vi "Decode NTC codes.vi"(11 "NTC Messages":T1(array[cluster])=[{"ID"=1808, "MSGTYPE"=0, "LEN"=8, "DATA[0]"=33, "DATA[1]"=11, "DATA[2]"=56, "DATA[3]"=1, "DATA[4]"=36, "DATA[5]"=0, "DATA[6]"=11, "DATA[7]"=0}, {"ID"=1808, "MSGTYPE"=0, "LEN"=8, "DATA[0]"=34, "DATA[1]"=1, "DATA[2]"=37, "DATA[3]"=0, "DATA[4]"=11, "DATA[5]"=0, "DATA[6]"=1, "DATA[7]"=64}, {"ID"=1808, "MSGTYPE"=0, "LEN"=8, "DATA[0]"=35, "DATA[1]"=0, "DATA[2]"=11, "DATA[3]"=0, "DATA[4]"=1, "DATA[5]"=68, "DATA[6]"=0, "DATA[7]"=11}, {"ID"=1808, "MSGTYPE"=0, "LEN"=8, "DATA[0]"=36, "DATA[1]"=0, "DATA[2]"=1, "DATA[3]"=73, "DATA[4]"=0, "DATA[5]"=11, "DATA[6]"=0, "DATA[7]"=1}, {"ID"=1808, "MSGTYPE"=0, "LEN"=8, "DATA[0]"=37, "DATA[1]"=80, "DATA[2]"=0, "DATA[3]"=11, "DATA[4]"=0, "DATA[5]"=1, "DATA[6]"=86, "DATA[7]"=0}, {"ID"=1808, "MSGTYPE"=0, "LEN"=8, "DATA[0]"=38, "DATA[1]"=11, "DATA[2]"=0, "DATA[3]"=1, "DATA[4]"=89, "DATA[5]"=0, "DATA[6]"=11, "DATA[7]"=0}, {"ID"=1808, "MSGTYPE"=0, "LEN"=8, "DATA[0]"=39, "DATA[1]"=1, "DATA[2]"=104, "DATA[3]"=0, "DATA[4]"=11, "DATA[5]"=0, "DATA[6]"=1, "DATA[7]"=105}, {"ID"=1808, "MSGTYPE"=0, "LEN"=8, "DATA[0]"=40, "DATA[1]"=0, "DATA[2]"=11, "DATA[3]"=0, "DATA[4]"=1, "DATA[5]"=114, "DATA[6]"=0, "DATA[7]"=11}, {"ID"=1808, "MSGTYPE"=0, "LEN"=8, "DATA[0]"=41, "DATA[1]"=0, "DATA[2]"=1, "DATA[3]"=115, "DATA[4]"=0, "DATA[5]"=11, "DATA[6]"=0, "DATA[7]"=1}, {"ID"=1808, "MSGTYPE"=0, "LEN"=8, "DATA[0]"=42, "DATA[1]"=144, "DATA[2]"=0, "DATA[3]"=11, "DATA[4]"=24, "DATA[5]"=1, "DATA[6]"=146, "DATA[7]"=0}, {"ID"=1808, "MSGTYPE"=0, "LEN"=8, "DATA[0]"=43, "DATA[1]"=11, "DATA[2]"=1, "DATA[3]"=0, "DATA[4]"=80, "DATA[5]"=2, "DATA[6]"=8, "DATA[7]"=0}, {"ID"=1808, "MSGTYPE"=0, "LEN"=8, "DATA[0]"=44, "DATA[1]"=0, "DATA[2]"=85, "DATA[3]"=2, "DATA[4]"=8, "DATA[5]"=0, "DATA[6]"=0, "DATA[7]"=176}, {"ID"=1808, "MSGTYPE"=0, "LEN"=8, "DATA[0]"=45, "DATA[1]"=2, "DATA[2]"=8, "DATA[3]"=0, "DATA[4]"=1, "DATA[5]"=96, "DATA[6]"=2, "DATA[7]"=73}, {"ID"=1808, "MSGTYPE"=0, "LEN"=8, "DATA[0]"=46, "DATA[1]"=0, "DATA[2]"=0, "DATA[3]"=0, "DATA[4]"=255, "DATA[5]"=0, "DATA[6]"=0, "DATA[7]"=0}] {"ID" format="%.0x"; "DATA[0]" format="%.0x"; "DATA[1]" format="%.0x"; "DATA[2]" format="%.0x"; "DATA[3]" format="%.0x"; "DATA[4]" format="%.0x"; "DATA[5]" format="%.0x"; "DATA[6]" format="%.0x"; "DATA[7]" format="%.0x"}) -> (2 "NTC codes":u32[](array[numeric]) format="%.0x", 3 "NTCs":string)   [LabVIEW 2025]
panel:
  out "NTC codes1":i32[](array[numeric])
  out "Parameters":i32[](array[numeric]) format="%.0x"
  out "s":i32[](array[numeric]) format="%.0x"
  out "a":i32[](array[numeric])
  out "NTC codes0":i32[](array[numeric]) format="%.0x"
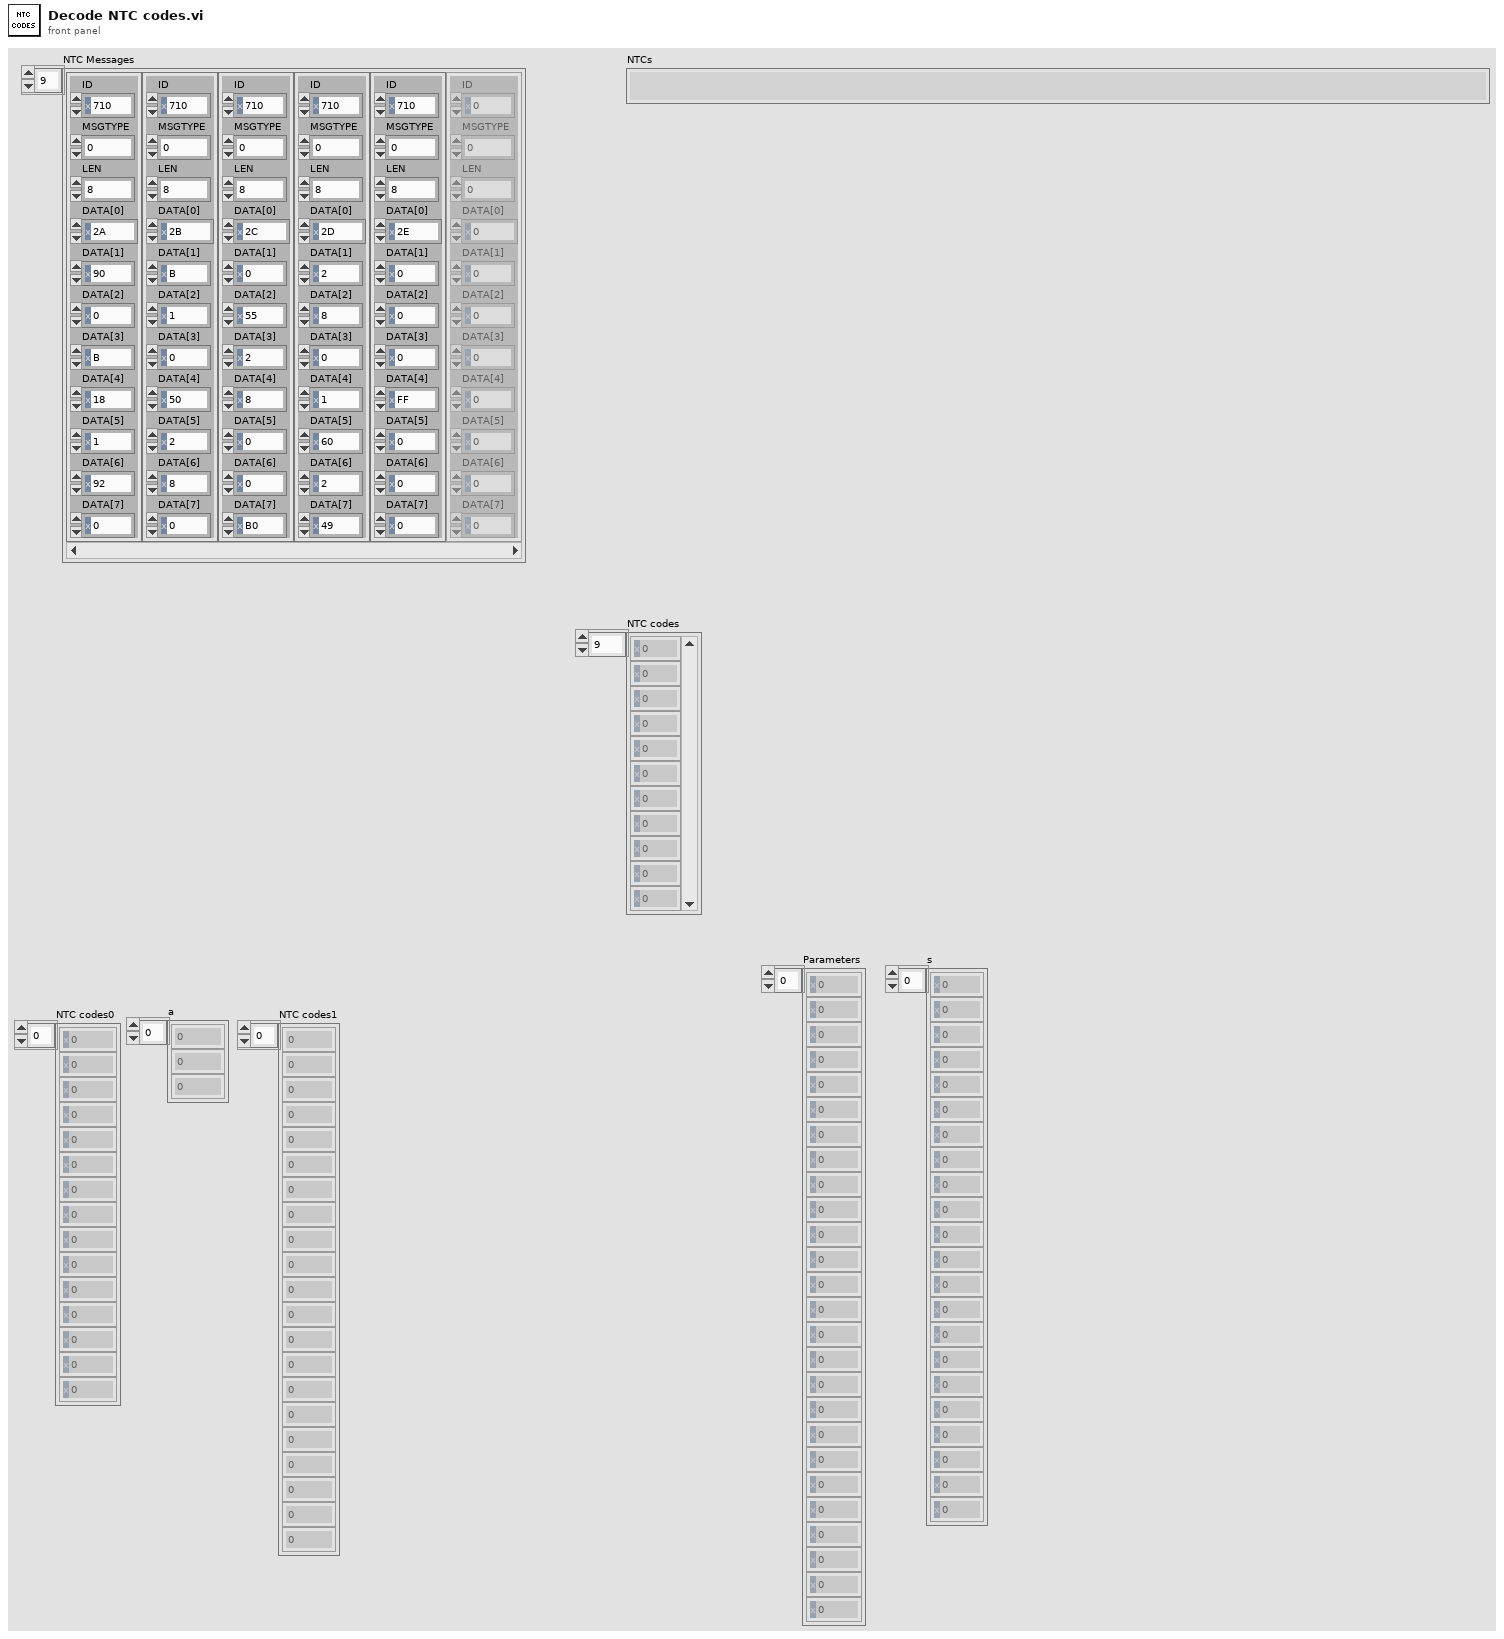
[diagram p1: front panel]
types:
  T1 = cluster{"ID":u32, "MSGTYPE":u8, "LEN":u8, "DATA[0]":u8, "DATA[1]":u8, "DATA[2]":u8, "DATA[3]":u8, "DATA[4]":u8, "DATA[5]":u8, "DATA[6]":u8, "DATA[7]":u8}[]
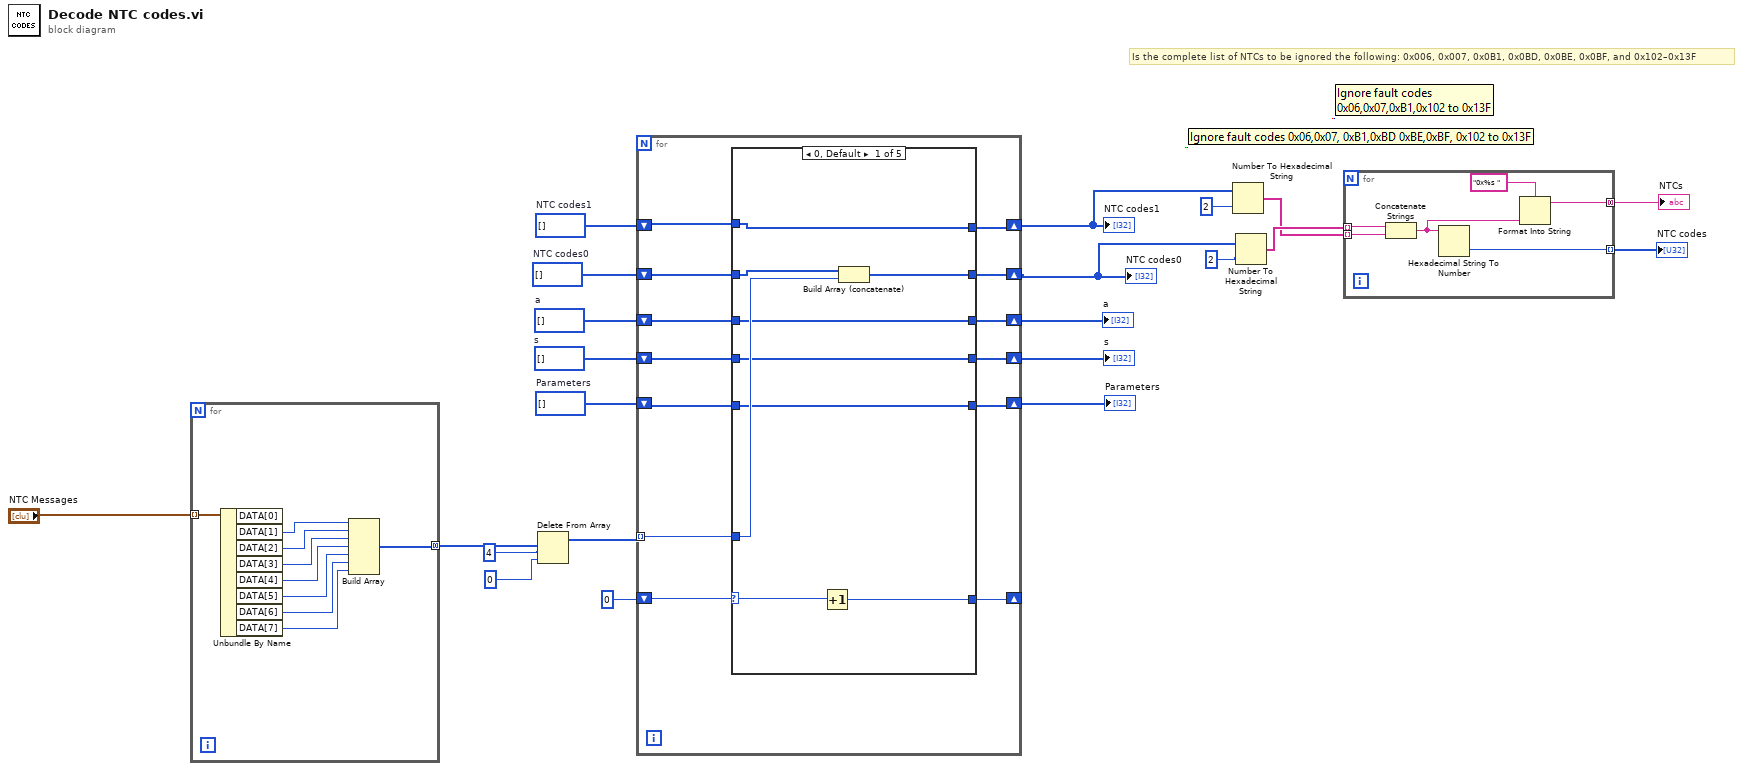
[diagram p0: block diagram]
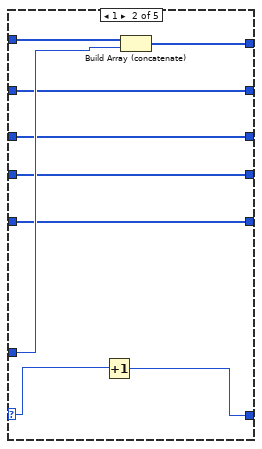
[diagram p2: hidden frame]
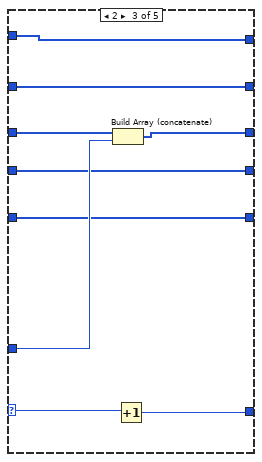
[diagram p3: hidden frame]
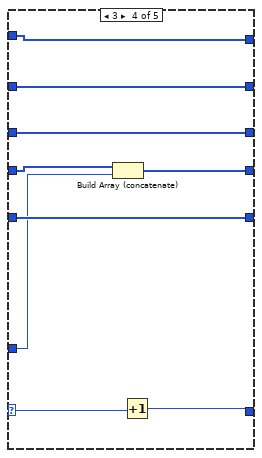
[diagram p4: hidden frame]
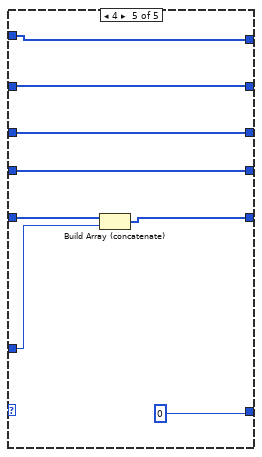
[diagram p5: hidden frame]
diagram:
  w13 = i32[] []  # NTC codes1
  w14 = i32[] []  # Parameters
  w15 = i32[] []  # s
  w16 = i32[] []  # a
  w17 = i32[] []  # NTC codes0
  # "Is the complete list of NTCs to be ignored the following: 0x006, 0x007, 0x0B1, 0x0BD, 0x0BE, 0x0BF, and 0x102–0x13F"
  n1 = for {
    tunnel: "NTC Messages" -> [w31] mode=indexing
    tunnel: [w23] -> w22 mode=concatenating
    n2 = Unbundle By Name(w31) -> ("DATA[1]"=w30:u8, "DATA[2]"=w29:u8, "DATA[3]"=w28:u8, "DATA[4]"=w27:u8, "DATA[5]"=w26:u8, "DATA[6]"=w25:u8, "DATA[7]"=w24:u8)  [unwired: 1 out]
    n3 = Build Array(w30, w29, w28, w27, w26, w25, w24) -> (w23:u8[])
  }
  n4 = Delete From Array(array=w22, length=4, index=0) -> (array with subset deleted=w19:u8[])  [unwired: 1 out]
  n5 = for {
    tunnel: w19 -> [w43] mode=indexing
    shift-right: [w34] -> _
    shift-left: 0 -> [w44]
    shift-right: [w41] -> w7
    shift-left: w17 -> [w42]
    shift-right: [w36] -> w10
    shift-left: w14 -> [w35]
    shift-right: [w37] -> w9
    shift-left: w15 -> [w38]
    shift-right: [w39] -> w11
    shift-left: w16 -> [w40]
    shift-right: [w32] -> w8
    shift-left: w13 -> [w33]
    n6 = case shown="0, Default" w44 {
      selector: w44 -> [w47 w59 w65 w74 _]
      tunnel: w43 -> [w52 w60 w68 w75 w82]
      tunnel: w42 -> [w53 w57 w71 w80 w88]
      tunnel: [w51 w57 w71 w80 w88] -> w41
      tunnel: w40 -> [w50 w56 w70 w79 w87]
      tunnel: [w50 w56 w69 w79 w87] -> w39
      tunnel: w38 -> [w49 w55 w67 w78 w86]
      tunnel: [w49 w55 w67 w77 w86] -> w37
      tunnel: [w48 w54 w66 w76 w83] -> w36
      tunnel: w35 -> [w48 w54 w66 w76 w84]
      tunnel: [w46 w58 w64 w73 0] -> w34
      tunnel: w33 -> [w45 w62 w63 w72 w81]
      tunnel: [w45 w61 w63 w72 w81] -> w32
      frame 0, Default {
        n7 = Increment(x=w47) -> (x+1=w46:i32)
        n8 = Build Array (concatenate)(w53, w52) -> (w51:i32[])
      }
      frame 1 {
        n9 = Increment(x=w59) -> (x+1=w58:i32)
        n10 = Build Array (concatenate)(w62, w60) -> (w61:i32[])
      }
      frame 2 {
        n11 = Build Array (concatenate)(w70, w68) -> (w69:i32[])
        n12 = Increment(x=w65) -> (x+1=w64:i32)
      }
      frame 3 {
        n13 = Build Array (concatenate)(w78, w75) -> (w77:i32[])
        n14 = Increment(x=w74) -> (x+1=w73:i32)
      }
      frame 4 {
        n15 = Build Array (concatenate)(w84, w82) -> (w83:i32[])
      }
    }
  }
  "NTC codes0" <- w7
  "a" <- w11
  "s" <- w9
  "Parameters" <- w10
  "NTC codes1" <- w8
  n16 = Number To Hexadecimal String(1:i16 2 ("width (-)"), 2:w8) -> (0:w5:string[])
  n17 = Number To Hexadecimal String(1:i16 2 ("width (-)"), 2:w7) -> (0:w6:string[])
  n18 = for {
    tunnel: w6 -> [w94] mode=indexing
    tunnel: w5 -> [w93] mode=indexing
    tunnel: [w92] -> w4 mode=indexing
    tunnel: [w89] -> w1 mode=concatenating
    n19 = Concatenate Strings(w94, w93) -> (w91:string)
    n20 = Hexadecimal String To Number(string=w91) -> (number=w92:u32)  [unwired: 2 in, 1 out]
    n21 = Format Into String(format string="0x%s ", w91) -> (resulting string=w89:string)  [unwired: 2 in, 1 out]
  }
  "NTC codes" <- w4
  "NTCs" <- w1
